vi "UsrProfiles-Window-Access pos.vi"(7 "Window Name":string, 9 "Access source":T1(ring), 11 "VI in":refnum<vi>) -> (0 "error out":errorcluster, 3 "VI out":refnum<vi>)   [LabVIEW 2013]
uses:
  Typedefs/Which path.ctl
  <vilib>/Utility/miscctls.llb/LVRectTypeDef.ctl
  <vilib>/Utility/config.llb/Read Key (String).vi
  <vilib>/Utility/config.llb/NI_LVConfig.lvlib
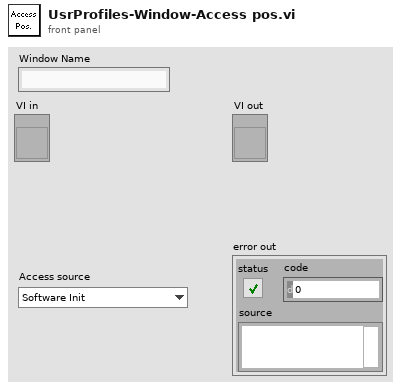
[diagram p1: front panel]
types:
  T1 = enum16{"Software Init", "User menu", "Switch User button"}
  T2 = enum32{"Invalid", "Standard", "Closed", "Hidden", "Minimized", "Maximized"}
  T3 = typedef "LVRectTypeDef.ctl" = cluster{"Left":i16, "Top":i16, "Right":i16, "Bottom":i16}
  T4 = typedef "Which path.ctl" = enum16{"Configuration Files", "Calibration Files", "Images", "Setup.ini", "Loaded User profile.ini", "User's-Previous session.ini", "New user profile.ini", "Selected User profile.ini", "User profiles folder", "Power meter scaling.txt", "FOV Cal.ini"}
  T5 = typedef "NI_LVConfig.lvlib/Config Data RefNum.ctl" = refnum<k1>
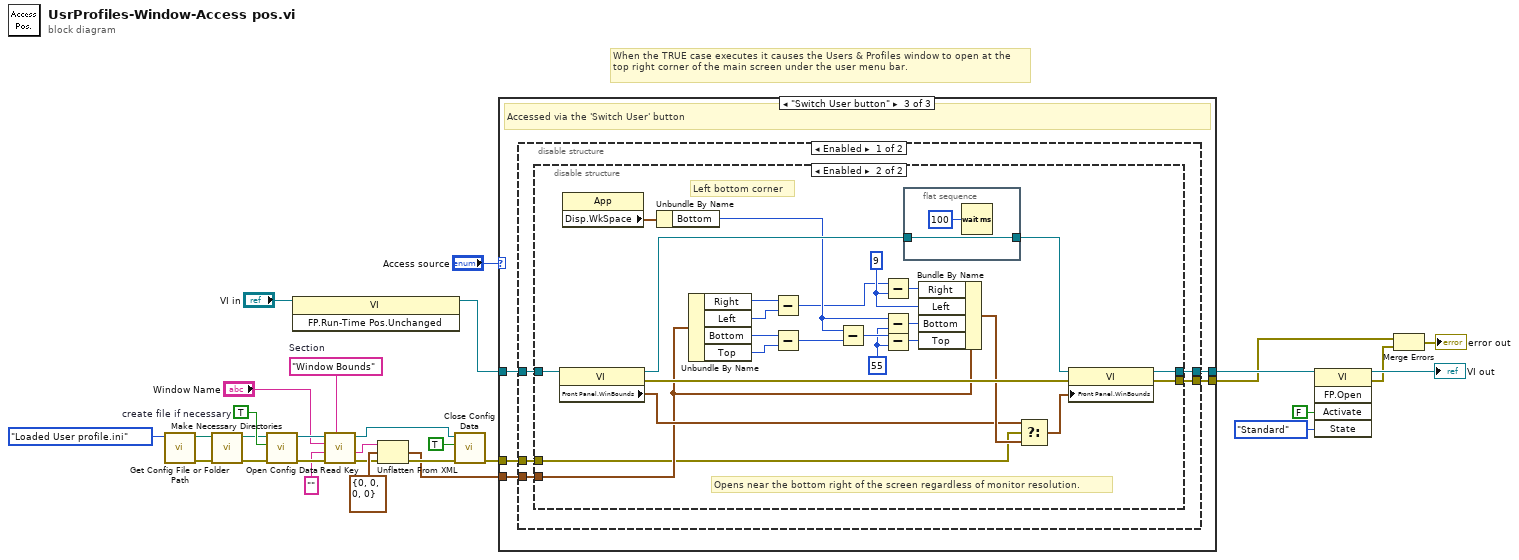
[diagram p0: block diagram]
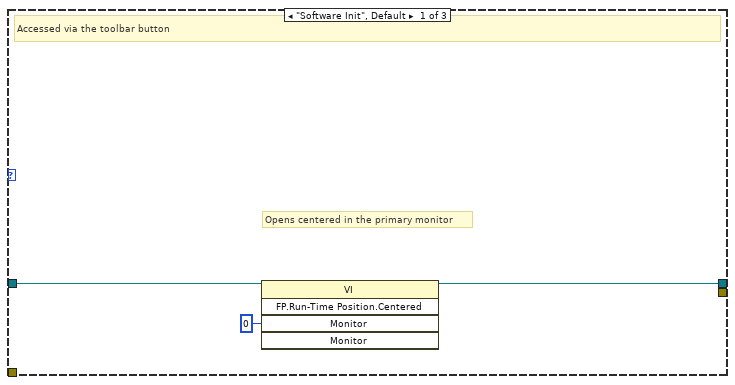
[diagram p2: hidden frame]
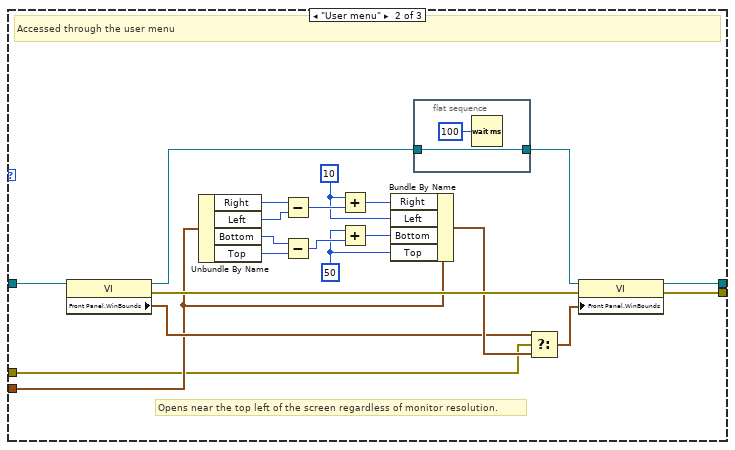
[diagram p3: hidden frame]
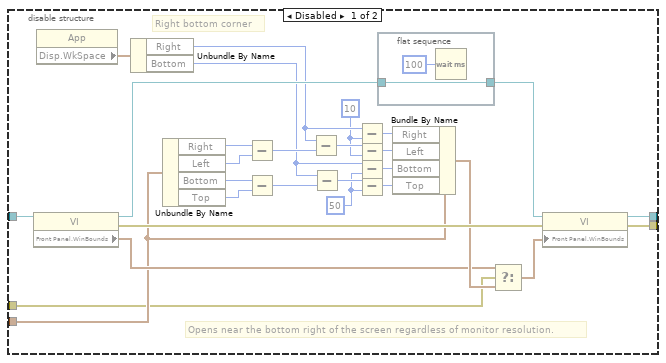
[diagram p4: hidden frame]
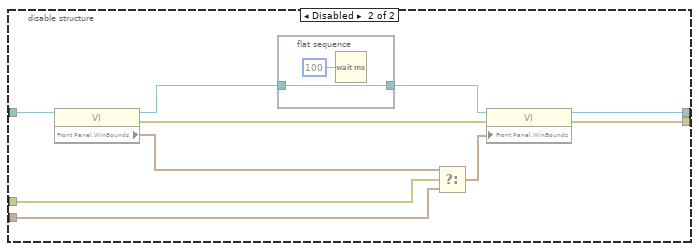
[diagram p5: hidden frame]
diagram:
  w13 = "Window Bounds"  # Section
  w17 = TRUE  # create file if necessary
  # "When the TRUE case executes it causes the Users & Profiles window to open at the top right corner of the main screen under the user menu bar."
  n1 = call "Get Config File or Folder Path.vi"("Which file or folder?"=Which_path."Loaded User profile.ini" ("Which path?")) -> ("Error Out"=w27:errorcluster, "File Path"=w14:path)  [unwired: 8 in, 1 out]
  n2 = call "Make Necessary Directories.vi"("error in"=w27, "Path"=w14) -> ("error out"=w25:errorcluster, "Duplicated path"=w16:path)  [unwired: 8 in]
  n3 = call <vilib>:"Open Config Data.vi"("error in (no error)"=w25, "create file if necessary (T)"=w17, "configuration file path"=w16) -> ("error out"=w23:errorcluster, "refnum"=w24:T5)  [unwired: 6 in, 1 out]
  n4 = invoke class="VI" method="FP.Run-Time Pos.Unchanged"(reference="VI in") -> (reference out=w4:refnum<vi>)  [unwired: 2 in, 2 out]
  n5 = call-poly <vilib>:"Read Key.vi"("section"=w13, "error in (no error)"=w23, "default value"="" ("xml string"), "key"="Window Name", "refnum"=w24) -> ("error out"=w19:errorcluster, "value"=w20:string, "refnum out"=w22:T5)  [unwired: 3 in, 1 out]
  n6 = Unflatten From XML(xml string=w20, type=T3 {"Left"=0, "Top"=0, "Right"=0, "Bottom"=0} ("Front Panel Window:Window Bounds"), error in (no error)=w19) -> (value=w11:T3, error out=w18:errorcluster)
  n7 = call <vilib>:"Close Config Data.vi"("error in (no error)"=w18, "write file if changed (T)"=TRUE ("write configuration file? (F)"), "refnum"=w22) -> ("error out"=w10:errorcluster)  [unwired: 7 in, 1 out]
  n8 = case shown="\"Switch User button\"" "Access source" {
    tunnel: w4 -> [w31 w51 w60]
    tunnel: [_ w50 w59] -> w3
    tunnel: [w30 w48 w58] -> w7
    tunnel: w11 -> [_ w34 w57]
    tunnel: w10 -> [_ w33 w56]
    frame "Software Init", Default {
      # "Opens centered in the primary monitor"
      # "Accessed via the toolbar button"
      n9 = invoke class="VI" method="FP.Run-Time Position.Centered"(reference=w31, "Monitor"=i16 0) -> (reference out=w30:refnum<vi>)  [unwired: 3 in, 4 out]
    }
    frame "User menu" {
      w35 = i16 50 ("Numeric")
      w36 = i16 10 ("Numeric")
      # "Opens near the top left of the screen regardless of monitor resolution."
      # "Accessed through the user menu"
      n10 = property on="Property Node" class="VI"(reference=w51) -> (reference out=w52:refnum<vi>, error out=w47:errorcluster, "Front Panel.WinBounds"=w39:T3)  [unwired: 1 in]
      n11 = Unbundle By Name(w34) -> ("Right"=w44:i16, "Left"=w46:i16, "Bottom"=w42:i16, "Top"=w45:i16)
      n12 = Subtract(x=w44, y=w46) -> (x-y=w43:i16)
      n13 = Subtract(x=w42, y=w45) -> (x-y=w38:i16)
      n14 = Add(x=w36, y=w43) -> (x+y=w37:i16)
      n15 = Add(x=w35, y=w38) -> (x+y=w41:i16)
      n16 = Bundle By Name(cluster=w34, "Right"=w37, "Left"=w36, "Bottom"=w41, "Top"=w35) -> (w40:T3)
      n17 = flat-sequence {
        tunnel: w52 -> [w54]
        tunnel: [w54] -> w53
        frame #0 {
          n18 = Wait (ms)(milliseconds to wait=u32 100) -> ()  [unwired: 1 out]
        }
      }
      n19 = Select(t=w39, s=w33, f=w40) -> (s? t:f=w49:T3)
      n20 = property on="Property Node" class="VI"(reference=w53, error in=w47, "Front Panel.WinBounds"=w49) -> (reference out=w48:refnum<vi>, error out=w50:errorcluster)
    }
    frame "Switch User button" {
      # "Accessed via the 'Switch User' button"
      n21 = disable-structure shown="Enabled" {
        disable-tunnel: w60 -> [w65 w127]
        disable-tunnel: [w64 w123] -> w59
        disable-tunnel: [w63 w124] -> w58
        disable-tunnel: w57 -> [w62 w125]
        disable-tunnel: w56 -> [w61 w126]
        frame Enabled {
          n22 = disable-structure shown="Enabled" {
            disable-tunnel: w65 -> [w91 w118]
            disable-tunnel: [w90 w117] -> w64
            disable-tunnel: [w88 w115] -> w63
            disable-tunnel: w62 -> [w80 w107]
            disable-tunnel: w61 -> [w79 w106]
            frame Disabled {
              w66 = i16 10 ("y")
              w67 = i16 50 ("y")
              # "Right bottom corner"
              # "Opens near the bottom right of the screen regardless of monitor resolution."
              n23 = property on="Property Node" class="VI"(reference=w91) -> (reference out=w92:refnum<vi>, error out=w87:errorcluster, "Front Panel.WinBounds"=w81:T3)  [unwired: 1 in]
              n24 = property on="Property Node" class="App"() -> ("Disp.WkSpace"=w78:T3)  [unwired: 2 in, 2 out]
              n25 = Unbundle By Name(w78) -> ("Right"=w74:i16, "Bottom"=w70:i16)
              n26 = Unbundle By Name(w80) -> ("Right"=w84:i16, "Left"=w86:i16, "Bottom"=w83:i16, "Top"=w85:i16)
              n27 = Subtract(x=w84, y=w86) -> (x-y=w77:i16)
              n28 = Subtract(x=w83, y=w85) -> (x-y=w76:i16)
              n29 = Subtract(x=w74, y=w77) -> (x-y=w73:i16)
              n30 = Subtract(x=w70, y=w76) -> (x-y=w69:i16)
              n31 = Subtract(x=w74, y=w66) -> (x-y=w75:i16)
              n32 = Subtract(x=w73, y=w66) -> (x-y=w72:i16)
              n33 = Subtract(x=w70, y=w67) -> (x-y=w71:i16)
              n34 = Subtract(x=w69, y=w67) -> (x-y=w68:i16)
              n35 = flat-sequence {
                tunnel: w92 -> [w94]
                tunnel: [w94] -> w93
                frame #0 {
                  n36 = Wait (ms)(milliseconds to wait=u32 100) -> ()  [unwired: 1 out]
                }
              }
              n37 = Bundle By Name(cluster=w80, "Right"=w75, "Left"=w72, "Bottom"=w71, "Top"=w68) -> (w82:T3)
              n38 = Select(t=w81, s=w79, f=w82) -> (s? t:f=w89:T3)
              n39 = property on="Property Node" class="VI"(reference=w93, error in=w87, "Front Panel.WinBounds"=w89) -> (reference out=w88:refnum<vi>, error out=w90:errorcluster)
            }
            frame Enabled {
              w97 = i16 9 ("y 2")
              w98 = i16 55 ("y")
              # "Left bottom corner"
              # "Opens near the bottom right of the screen regardless of monitor resolution."
              n40 = property on="Property Node" class="VI"(reference=w118) -> (reference out=w119:refnum<vi>, error out=w114:errorcluster, "Front Panel.WinBounds"=w108:T3)  [unwired: 1 in]
              n41 = property on="Property Node" class="App"() -> ("Disp.WkSpace"=w105:T3)  [unwired: 2 in, 2 out]
              n42 = Unbundle By Name(w105) -> ("Bottom"=w101:i16)
              n43 = Unbundle By Name(w107) -> ("Right"=w111:i16, "Left"=w113:i16, "Bottom"=w110:i16, "Top"=w112:i16)
              n44 = Subtract(x=w111, y=w113) -> (x-y=w96:i16)
              n45 = Subtract(x=w110, y=w112) -> (x-y=w104:i16)
              n46 = Subtract(x=w101, y=w104) -> (x-y=w100:i16)
              n47 = Subtract(x=w96, y=w97) -> (x-y=w103:i16)
              n48 = Subtract(x=w101, y=w98) -> (x-y=w102:i16)
              n49 = Subtract(x=w100, y=w98) -> (x-y=w99:i16)
              n50 = flat-sequence {
                tunnel: w119 -> [w121]
                tunnel: [w121] -> w120
                frame #0 {
                  n51 = Wait (ms)(milliseconds to wait=u32 100) -> ()  [unwired: 1 out]
                }
              }
              n52 = Bundle By Name(cluster=w107, "Right"=w103, "Left"=w97, "Bottom"=w102, "Top"=w99) -> (w109:T3)
              n53 = Select(t=w108, s=w106, f=w109) -> (s? t:f=w116:T3)
              n54 = property on="Property Node" class="VI"(reference=w120, error in=w114, "Front Panel.WinBounds"=w116) -> (reference out=w115:refnum<vi>, error out=w117:errorcluster)
            }
          }
        }
        frame Disabled {
          n55 = property on="Property Node" class="VI"(reference=w127) -> (reference out=w129:refnum<vi>, error out=w131:errorcluster, "Front Panel.WinBounds"=w132:T3)  [unwired: 1 in]
          n56 = flat-sequence {
            tunnel: w129 -> [w133]
            tunnel: [w133] -> w128
            frame #0 {
              n57 = Wait (ms)(milliseconds to wait=u32 100) -> ()  [unwired: 1 out]
            }
          }
          n58 = Select(t=w132, s=w126, f=w125) -> (s? t:f=w130:T3)
          n59 = property on="Property Node" class="VI"(reference=w128, error in=w131, "Front Panel.WinBounds"=w130) -> (reference out=w124:refnum<vi>, error out=w123:errorcluster)
        }
      }
    }
  }
  n60 = invoke class="VI" method="FP.Open"(reference=w7, "Activate"=FALSE ("Activate?"), "State"=T2."Standard" ("Front Panel Window:State")) -> (reference out=→"VI out":refnum<vi>, error out=w2:errorcluster)  [unwired: 2 in, 3 out]
  n61 = Merge Errors(w3, w2) -> (→"error out":errorcluster)
